vi "CreateTimeVector.vi"(7 "Sampling Frequency":dbl=1.0, 11 "Array in":dbl[](array[numeric])) -> (3 "Array out":dbl[](array[numeric]))   [LabVIEW 2013, in "main.lvlib"]
uses:
  main.lvlib
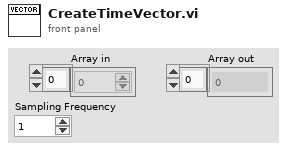
[diagram p1: front panel]
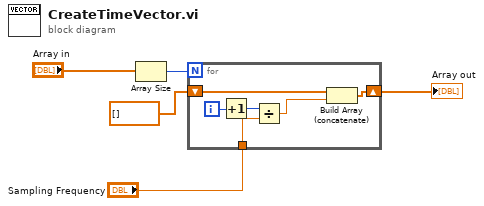
[diagram p0: block diagram]
diagram:
  n1 = Array Size(array="Array in") -> (size(s)=w3:i32)
  n2 = for {
    N: w3 -> [_]
    shift-right: [w7] -> w1
    shift-left: dbl[] [] -> [w11]
    tunnel: "Sampling Frequency" -> [w8]
    i -> [w10]
    n3 = Increment(x=w10) -> (x+1=w9:i32)
    n4 = Divide(x=w9, y=w8) -> (x/y=w6:dbl)
    n5 = Build Array (concatenate)(w11, w6) -> (w7:dbl[])
  }
  "Array out" <- w1
